vi "niRFUtil FWK Parse Option String.vi"(6 "Remove Tag?":bool, 8 "error in (no error)":errorcluster, 9 "Tag Name":string, 10 "Property Name":string, 11 "Option String":string) -> (0 "error out":errorcluster, 1 "Tag Available?":bool, 2 "Tag Value":string, 3 "Parsed String":string)   [LabVIEW 2015, in "niRFUtil.lvlib"]
doc: "This VI will Parse the incoming Option String and gives out the required Tag Value. \nBy enabling \"Remove Tag?\" Flag this VI will remove the inputted Tag and its value from the Option string. If it is not Enabled Only Tag value will be extracted and Option String will be same as inputted."
uses:
  niRFUtil.lvlib
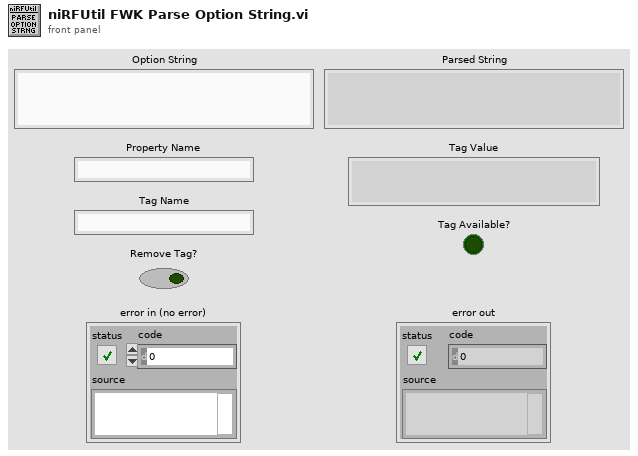
[diagram p1: front panel]
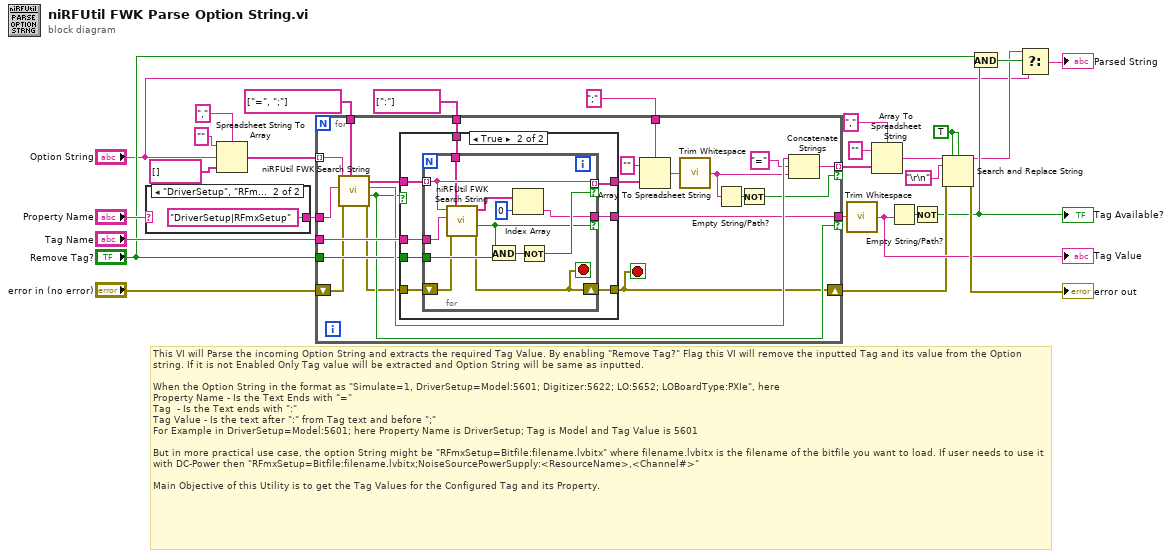
[diagram p0: block diagram]
diagram:
  w12 = TRUE ("replace all? (F)")
  # "This VI will Parse the incoming Option String and extracts the required Tag Value. By enabling \"Remove Tag?\" Flag this VI will remove the inputted Tag and its value from the Option string. If it is not Enabled Only Tag value will be extracted and Option String will be same as inputted.\n\nWhen the Option String in the format as \"Simulate=1, DriverSetup=Model:5601; Digitizer:5622; LO:5652; LOBoardType:PXIe\", here\nProperty Name - Is the Text Ends with \"=\"\nTag  - Is the Text ends with \":\"\nTag Value - Is the text after \":\" from Tag text and before \";\" \nFor Example in DriverSetup=Model:5601; here Property Name is DriverSetup; Tag is Model and Tag Value is 5601\n\nBut in more practical use case, the option String might be \"RFmxSetup=Bitfile:filename.lvbitx\" where filename.lvbitx is the filename of the bitfile you want to load. If user needs to use it with DC-Power then \"RFmxSetup=Bitfile:filename.lvbitx;NoiseSourcePowerSupply:<ResourceName>,<Channel#>\"\n\nMain Objective of this Utility is to get the Tag Values for the Configured Tag and its Property."
  n1 = case shown="\"DriverSetup\", \"RFmxSetup\"" "Property Name" {
    selector: "Property Name" -> [w29 _]
    tunnel: [w29 "DriverSetup|RFmxSetup" ("Property Name")] -> w18
    frame Default {
    }
    frame "DriverSetup", "RFmxSetup" {
    }
  }
  n2 = Spreadsheet String To Array(delimiter (Tab)=",", format string="", spreadsheet string="Option String", array type (2D Dbl)=string[] []) -> (array=w20:string[])
  n3 = for {
    tunnel: w20 -> [w40] mode=indexing
    tunnel: string[] ["=", ";"] ("Delimiters") -> [w41]
    tunnel: "Tag Name" -> [w51]
    tunnel: "Remove Tag?" -> [w45]
    tunnel: ";" ("delimiter (Tab)") -> [w48]
    tunnel: [w47] -> w16 mode=indexing if=w32
    tunnel: w18 -> [w38]
    tunnel: [w44] -> w8 if=w43
    tunnel: string[] [":"] ("Delimiters") -> [w39]
    shift-right: [w31] -> w7
    shift-left: "error in (no error)" -> [w37]
    stop <- w31 stop-if-true
    n4 = call "niRFUtil FWK Search String.vi"("Delimiters"=w41, "error in"=w37, "Search String"=w38, "Input String"=w40) -> ("error out"=w36:errorcluster, "Whole Word Matched?"=w43:bool, "Found String"=w46:string, "Remaining String"=w52:string[])  [unwired: 4 in]
    n5 = case shown="True" w43 {
      tunnel: w52 -> [w54 w62]
      tunnel: w51 -> [_ w61]
      tunnel: [w54 w59] -> w50
      tunnel: w45 -> [_ w60]
      tunnel: [_ w58] -> w44
      tunnel: w39 -> [_ w57]
      tunnel: w36 -> [w53 w56]
      tunnel: [w53 w55] -> w31
      frame False {
      }
      frame True {
        n6 = for {
          tunnel: w62 -> [w71] mode=indexing
          tunnel: w61 -> [w68]
          tunnel: [w71] -> w59 mode=indexing if=w73
          tunnel: w60 -> [w74]
          tunnel: [w63] -> w58 if=w69
          tunnel: w57 -> [w70]
          shift-right: [w66] -> w55
          shift-left: w56 -> [w67]
          stop <- w66 stop-if-true
          n7 = call "niRFUtil FWK Search String.vi"("Delimiters"=w70, "error in"=w67, "Search String"=w68, "Input String"=w71) -> ("error out"=w66:errorcluster, "Whole Word Matched?"=w69:bool, "Remaining String"=w65:string[])  [unwired: 4 in, 1 out]
          n8 = And(x=w69, y=w74) -> (x .and. y?=w72:bool)
          n9 = Index Array(array=w65, index=0) -> (element=w63:string)
          n10 = Not(x=w72) -> (.not. x?=w73:bool)
        }
      }
    }
    n11 = Array To Spreadsheet String(delimiter (Tab)=w48, array=w50, 3:"" ("format string")) -> (spreadsheet string=w42:string)
    n12 = call <vilib>:"Trim Whitespace.vi"("string"=w42) -> ("trimmed string"=w35:string)  [unwired: 1 in]
    n13 = Empty String/Path?(string/path=w35) -> (empty?=w33:bool)
    n14 = Not(x=w33) -> (.not. x?=w32:bool)
    n15 = Concatenate Strings(w46, "=" ("string"), w35) -> (w47:string)
  }
  n16 = call <vilib>:"Trim Whitespace.vi"("string"=w8) -> ("trimmed string"=w24:string)  [unwired: 1 in]
  "Tag Value" <- w24
  n17 = Array To Spreadsheet String(delimiter (Tab)=",", array=w16, 3:"" ("format string")) -> (spreadsheet string=w13:string)
  n18 = Empty String/Path?(string/path=w24) -> (empty?=w9:bool)
  n19 = Not(x=w9) -> (.not. x?=w6:bool)
  "Tag Available?" <- w6
  n20 = Search and Replace String(replace all?=w12, case sensitive?=w12, input string=w13, search string="\r\n", error in=w7) -> (result string=w3:string, error out=→"error out":errorcluster)  [unwired: 3 in, 2 out]
  n21 = And(x="Remove Tag?", y=w6) -> (x .and. y?=w4:bool)
  n22 = Select(t=w3, s=w4, f="Option String") -> (s? t:f=→"Parsed String":string)
